vi "Actor Core.vi"(8 "error in":errorcluster, 11 "Analog Reader in":refnum<class "Analog Reader.lvclass">) -> (0 "error out":errorcluster, 3 "Actor out":refnum<class "Actor.lvclass">)   [LabVIEW 2024, in "DAQmx Actor.lvlib" / "Analog Reader.lvclass"]
doc: "<p>(<strong>Filename</strong>: <span class=\"dnl\">Actor Framework.lvlib:Actor.lvclass:Actor Core.vi</span>)</p>\n<p>Receives messages to the actor, reacts to them, and initiates any error handling that may shut the actor down.</p>\n<p>Descendant classes may override this VI to append parallel tasks for the actor to complete while it handles messages. Overrides use the <a href=\"nihelplauncher://docs/csh?context=lvcore_glang_udclass\">Call Parent Class Method</a> node.</p>"
uses:
  Analog Reader.lvclass
  <vilib>/ActorFramework/Actor/Actor.lvclass
  <vilib>/ActorFramework/Actor/Actor.lvclass/Actor.ctl
  <vilib>/ActorFramework/Message Enqueuer/Message Enqueuer.lvclass/Message Enqueuer.ctl
  Analog Reader.lvclass/Analog Reader.ctl
  Analog Reader Messages/Analog Input Data Msg/Analog Input Data Msg.lvclass/Analog Input Data Msg.ctl
  <vilib>/ActorFramework/Message Enqueuer/Init from Existing Queue.vi
  <vilib>/ActorFramework/Message Enqueuer/Enqueue.vi
  Analog Reader Messages/Analog Input Data Msg/Analog Input Data Msg.lvclass
  <vilib>/ActorFramework/Message Priority Queue/Priority Enqueue.vi
  <vilib>/DAQmx/miscellaneous.llb/DAQmx Fill In Error Info.vi
  <vilib>/ActorFramework/Message Enqueuer/Message Enqueuer.lvclass
  <vilib>/DAQmx/read.llb/DAQmx Read (Analog 1D Wfm NChan NSamp).vi
  DAQmx Actor/DAQmx Actor.lvclass
  Analog Reader Helper/Analog Reader Helper.lvclass
  C:/Users/uspoaotto/OneDrive - Oregon Tool/Desktop/working copies/DAQmxActor/src/DAQmx Actor/DAQmx Actor/DAQmx Actor.lvclass
  C:/Program Files (x86)/National Instruments/LabVIEW 2024/vi.lib/ActorFramework/Actor/Actor.lvclass
  C:/Users/uspoaotto/OneDrive - Oregon Tool/Desktop/working copies/DAQmxActor/src/DAQmx Actor/Analog Reader/Analog Reader.lvclass
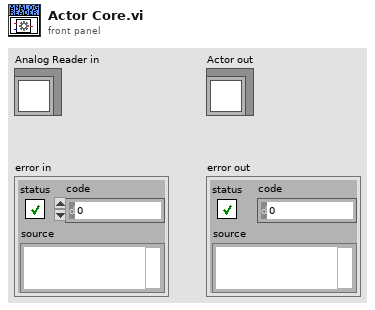
[diagram p1: front panel]
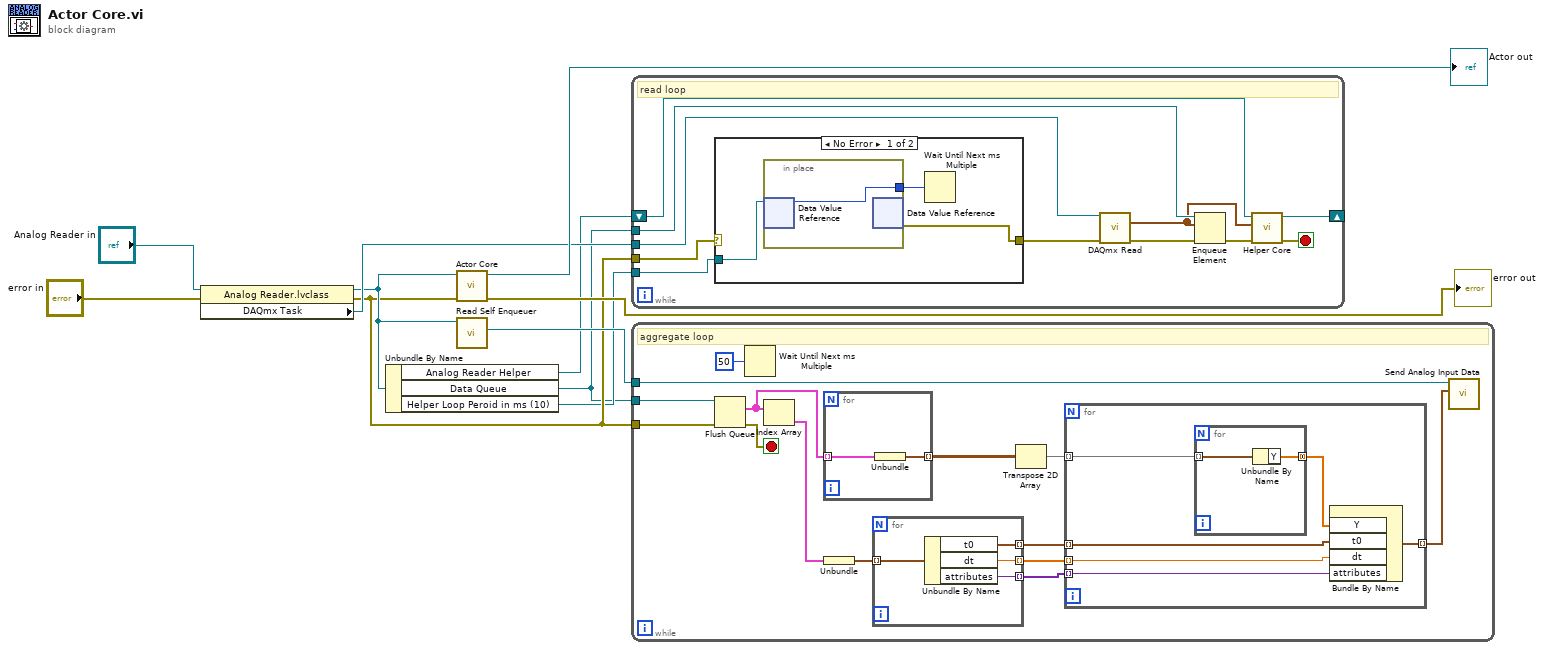
[diagram p0: block diagram]
diagram:
  n1 = property class="Analog Reader.lvclass"(reference="Analog Reader in", error in="error in") -> (reference out=w5:refnum<class "Analog Reader.lvclass">, error out=w4:errorcluster, "DAQmx Task"=w7:refnum<k21>)
  n2 = Unbundle By Name(w5) -> ("Analog Reader Helper"=w3:refnum<class "Analog Reader Helper.lvclass">, "Data Queue"=w1:refnum<queue>, "Helper Loop Peroid in ms (10)"=w2:refnum<data-value>)
  n3 = call-parent "Actor Core.vi"("error in"=w4, "Actor in"=w5) -> ("error out"=→"error out":errorcluster, "Actor out"=→"Actor out":refnum<class "Actor.lvclass">)  [unwired: 8 in]
  n4 = call <vilib>:"Read Self Enqueuer.vi"("Actor"=w5) -> ("Self Enqueuer"=w6:refnum<class "Message Enqueuer.lvclass">)  [unwired: 10 in]
  n5 = while {
    tunnel: w7 -> [w22]
    tunnel: w4 -> [w12]
    tunnel: w1 -> [w21]
    shift-right: [w16] -> _
    shift-left: w3 -> [w15]
    tunnel: w2 -> [w14]
    stop <- w17 stop-if-true
    # "read loop"
    n6 = case shown="No Error" w12 {
      selector: w12 -> [_ w27]
      tunnel: w14 -> [w25 _]
      tunnel: [w24 w27] -> w13
      frame No Error {
        n7 = in-place {
          in-place-border: [w26] -> w23
          n8 = in-place-dvr #1(w25) -> (w26:i32)  [unwired: 1 out]
          n9 = in-place-dvr #1() -> (w24:errorcluster)  [unwired: 1 in, 1 out]
        }
        n10 = Wait Until Next ms Multiple(millisecond multiple=w23) -> ()  [unwired: 1 out]
      }
      frame Error {
      }
    }
    n11 = call-poly <vilib>:"DAQmx Read.vi"("task/channels in"=w22, "error in"=w13) -> ("data"=w19:waveform(dbl)[], "error out"=w20:errorcluster)  [unwired: 11 in, 1 out]
    n12 = Enqueue Element(queue=w21, element=w19, error in (no error)=w20) -> (error out=w18:errorcluster)  [unwired: 1 in, 2 out]
    n13 = call-dynamic "Helper Core.vi"("error in (no error)"=w18, "data"=w19, "Analog Reader Helper in"=w15) -> ("error out"=w17:errorcluster, "Analog Reader Helper out"=w16:refnum<class "Analog Reader Helper.lvclass">)  [unwired: 7 in]
  }
  n14 = while {
    tunnel: w4 -> [w39]
    tunnel: w1 -> [w40]
    tunnel: w6 -> [w28]
    stop <- w30 stop-if-true
    # "aggregate loop"
    n15 = Flush Queue(queue=w40, error in (no error)=w39) -> (remaining elements=w33:cluster{waveform(dbl)[]}[], error out=w30:errorcluster)  [unwired: 1 out]
    n16 = Wait Until Next ms Multiple(millisecond multiple=u32 50) -> ()  [unwired: 1 out]
    n17 = Index Array(array=w33) -> (element=w32:cluster{waveform(dbl)[]})  [unwired: 1 in]
    n18 = for {
      tunnel: w33 -> [w55] mode=indexing
      tunnel: [w54] -> w34 mode=indexing
      n19 = Unbundle(w55) -> (w54:waveform(dbl)[])
    }
    n20 = Unbundle(w32) -> (w31:waveform(dbl)[])
    n21 = for {
      tunnel: w31 -> [w45] mode=indexing
      tunnel: [w44] -> w37 mode=indexing
      tunnel: [w43] -> w36 mode=indexing
      tunnel: [w42] -> w35 mode=indexing
      n22 = Unbundle By Name(w45) -> ("t0"=w44:timestamp, "dt"=w43:dbl, "attributes"=w42:variant)
    }
    n23 = Transpose 2D Array(2D array=w34) -> (transposed array=w38:waveform(dbl)[][])
    n24 = for {
      tunnel: w38 -> [w51] mode=indexing
      tunnel: [w50] -> w29 mode=indexing
      tunnel: w37 -> [w48] mode=indexing
      tunnel: w36 -> [w47] mode=indexing
      tunnel: w35 -> [w46] mode=indexing
      n25 = for {
        tunnel: w51 -> [w53] mode=indexing
        tunnel: [w52] -> w49 mode=concatenating
        n26 = Unbundle By Name(w53) -> ("Y"=w52:dbl[])
      }
      n27 = Bundle By Name("Y"=w49, "t0"=w48, "dt"=w47, "attributes"=w46) -> (w50:waveform(dbl))  [unwired: 1 in]
    }
    n28 = call "Send Analog Input Data.vi"("Analog Input Data"=w29, "Message Enqueuer"=w28) -> ()  [unwired: 8 in, 2 out]
  }
